vi "ExProg_InitScriptState.vi"() -> (3 "Script exec state out":T1)   [LabVIEW 2011]
uses:
  ExProgState.ctl
  Motors/MotorPosType.ctl
  Typedefs/XYf.ctl
  GlobalVariables.vi
panel:
  in  "Script exec state in (constant)":T1={"Wanted Motorpos"={"Magnet Z"=24.5544, "Magnet rotation"=18.99, "Camera"={"X"=0.0, "Y"=0.0}, "Piezo XY"={"X"=0.0, "Y"=0.0}, "Piezo Z"=54.9963}, "Goal motorpos"={"Magnet Z"=20.0, "Magnet rotation"=80.0, "Camera"={"X"=0.0, "Y"=0.0}, "Piezo XY"={"X"=0.0, "Y"=0.0}, "Piezo Z"=54.996}, "Instruction"=2, "Speed"={"Magnet Z"=0.0, "Magnet rotation"=0.0, "Camera"={"X"=0.0, "Y"=0.0}, "Piezo XY"={"X"=0.0, "Y"=0.0}, "Piezo Z"=0.0}, "New instruction?"=FALSE, "Instruction start time"=0.0}
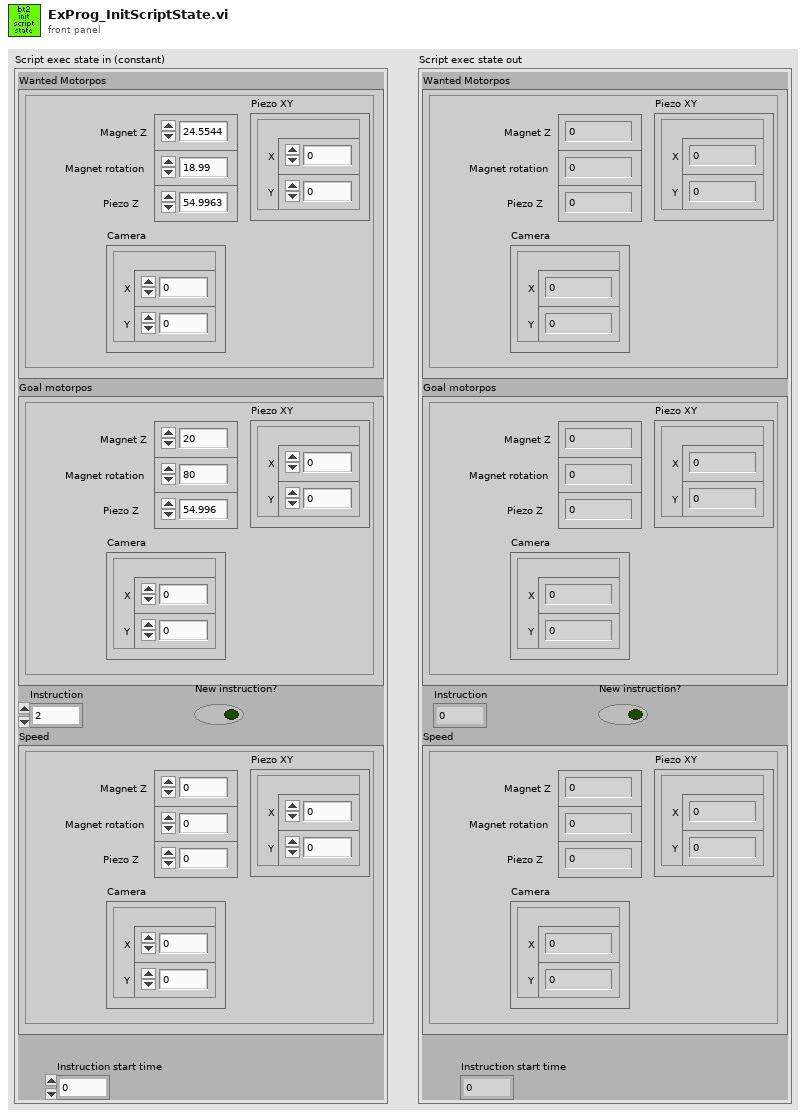
[diagram p1: front panel]
types:
  T1 = typedef "ExProgState.ctl" = cluster{"Wanted Motorpos":T2, "Goal motorpos":T2, "Instruction":i32, "Speed":T2, "New instruction?":bool, "Instruction start time":dbl}
  T2 = typedef "MotorPosType.ctl" = cluster{"Magnet Z":dbl, "Magnet rotation":dbl, "Camera":T3, "Piezo XY":T3, "Piezo Z":dbl}
  T3 = typedef "XYf.ctl" = cluster{"X":sgl, "Y":sgl}
  T4 = typedef "MotorStateType.ctl" = cluster{"Enabled?":bool, "Current Position":T2, "Update counter":i32}
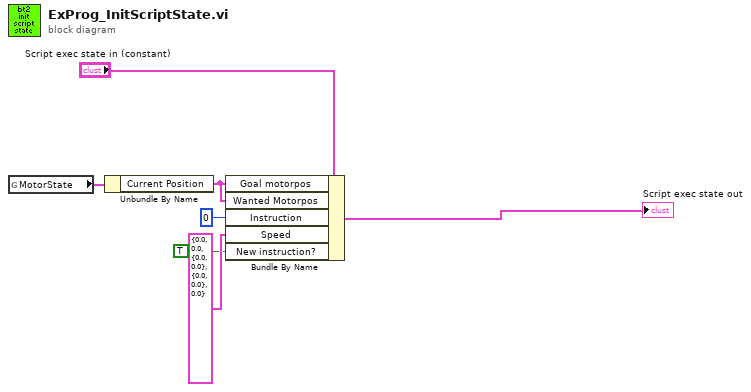
[diagram p0: block diagram]
diagram:
  n1 = global read "GlobalVariables.vi" "MotorState"() -> (w2:T4)
  n2 = Unbundle By Name(w2) -> ("Current Position"=w3:T2)
  n3 = Bundle By Name(cluster="Script exec state in (constant)", "Goal motorpos"=w3, "Wanted Motorpos"=w3, "Instruction"=0, "Speed"=T2 {"Magnet Z"=0.0, "Magnet rotation"=0.0, "Camera"={"X"=0.0, "Y"=0.0}, "Piezo XY"={"X"=0.0, "Y"=0.0}, "Piezo Z"=0.0}, "New instruction?"=TRUE) -> (→"Script exec state out":T1)
